vi "ForceAndPressureAhmed.vi"() -> ()   [LabVIEW 2017]
uses:
  <vilib>/Analysis/Matrix/Numeric/Conversions/Matrix To Array - RM.vi
  <vilib>/Analysis/NI_AALBase.lvlib
  <vilib>/Analysis/Matrix/NI_Matrix.lvlib
panel:
  out "Velocity (m/s)":dbl=1.0208025474683848
  out "Force Mean Convergence":dbl(graph)=0.23332198796908798
  out "Pressure Mean Convergence":dbl(graph)=0.00022051026462577283
  in  "Balance Check":i32
  in  "Tapping Check":i32=1
  in  "Comment":string="test"
  in  "Time (s)":dbl=10.0 format="%#_13g"
  in  "Frequency (Hz)":dbl=1000.0 format="%#_13g"
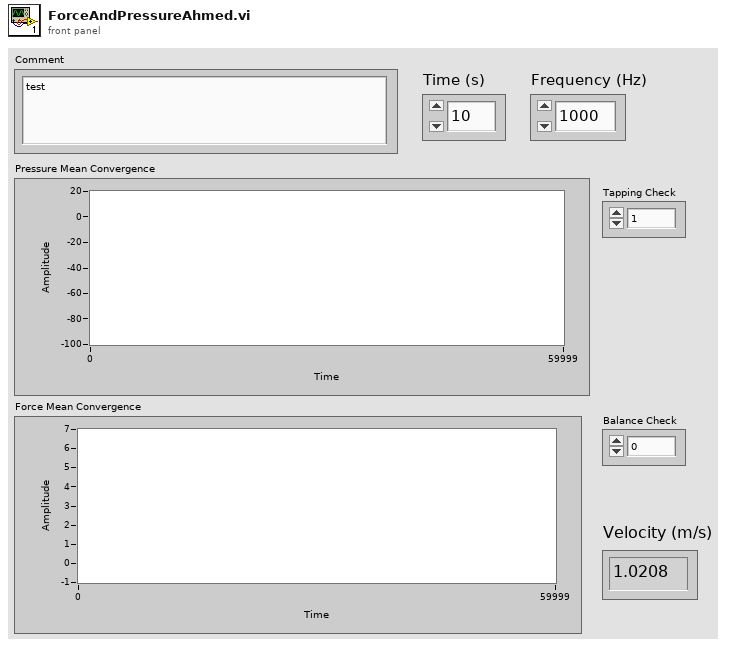
[diagram p1: front panel]
types:
  T1 = typedef "Real Matrix NI_Silver.ctl" = dbl[][]
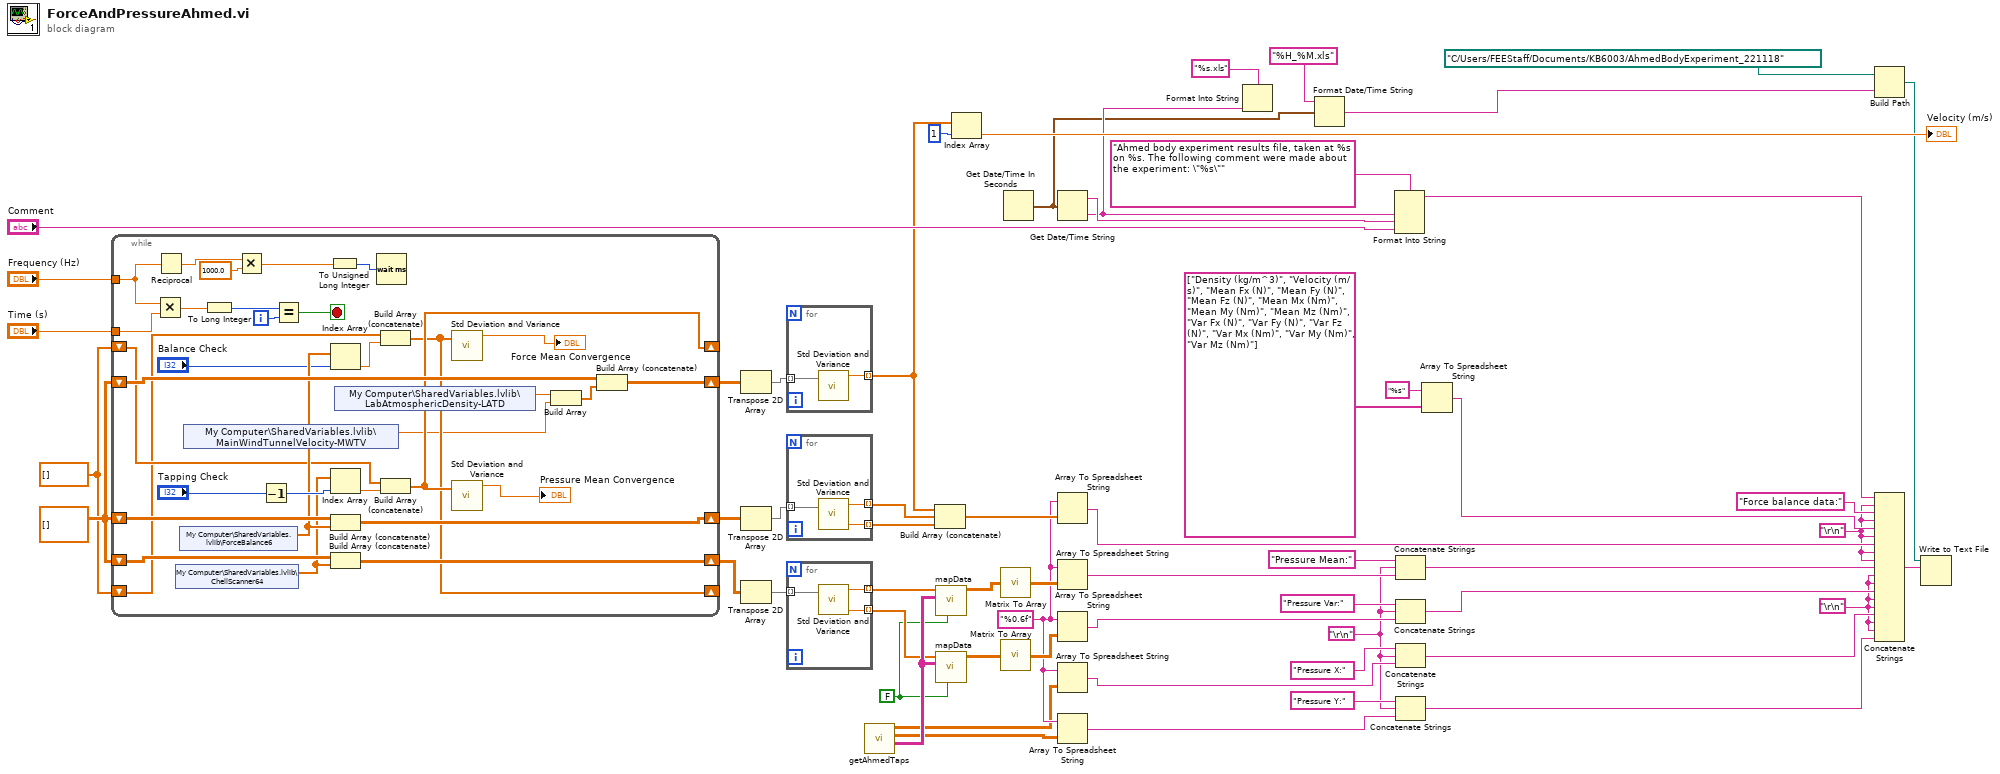
[diagram p0: block diagram]
diagram:
  w15 = dbl[] []
  w20 = "\r\n"
  w24 = "\r\n"
  w12 = "\r\n"
  w35 = "%0.6f" ("format string")
  w50 = FALSE ("Zero Index")
  w46 = dbl[][] []
  n1 = while {
    tunnel: "Frequency (Hz)" -> [w87]
    tunnel: "Time (s)" -> [w86]
    shift-right: [w81] -> w57
    shift-left: w46 -> [w80]
    shift-right: [w82] -> w56
    shift-left: w46 -> [w79]
    shift-right: [w76] -> w45
    shift-left: w46 -> [w75]
    shift-right: [w68] -> _
    shift-left: w15 -> [w70]
    shift-right: [w64] -> _
    shift-left: w15 -> [w66]
    i -> [w69]
    stop <- w83 stop-if-true
    n2 = Multiply(x=w87, y=w86) -> (x*y=w85:dbl)
    n3 = Reciprocal(x=w87) -> (1/x=w91:dbl)
    n4 = shared-variable "My Computer\\SharedVariables.lvlib\\ChellScanner64"() -> (w61:dbl[])  [unwired: 1 in, 1 out]
    n5 = shared-variable "My Computer\\SharedVariables.lvlib\\ForceBalance6"() -> (w72:dbl[])  [unwired: 1 in, 1 out]
    n6 = shared-variable "My Computer\\SharedVariables.lvlib\\MainWindTunnelVelocity-MWTV"() -> (w60:dbl)  [unwired: 1 in, 1 out]
    n7 = To Long Integer(number=w85) -> (32bit integer=w84:i32)
    n8 = Multiply(x=w91, y=1000.0) -> (x*y=w90:dbl)
    n9 = Decrement(x="Tapping Check") -> (x-1=w73:i32)
    n10 = Equal?(x=w84, y=w69) -> (x = y?=w83:bool)
    n11 = To Unsigned Long Integer(number=w90) -> (unsigned 32bit integer=w89:u32)
    n12 = Index Array(array=w72, index="Balance Check") -> (element=w65:dbl)
    n13 = Index Array(array=w61, index=w73) -> (element=w62:dbl)
    n14 = Build Array (concatenate)(w80, w72) -> (w81:dbl[][])
    n15 = Build Array (concatenate)(w79, w61) -> (w82:dbl[][])
    n16 = shared-variable "My Computer\\SharedVariables.lvlib\\LabAtmosphericDensity-LATD"() -> (w78:dbl)  [unwired: 1 in, 1 out]
    n17 = Wait (ms)(milliseconds to wait=w89) -> ()  [unwired: 1 out]
    n18 = Build Array (concatenate)(w66, w65) -> (w64:dbl[])
    n19 = Build Array (concatenate)(w70, w62) -> (w68:dbl[])
    n20 = call <vilib>:"Std Deviation and Variance.vi"("X"=w64) -> ("mean"=→"Force Mean Convergence":dbl)  [unwired: 1 in, 2 out]
    n21 = call <vilib>:"Std Deviation and Variance.vi"("X"=w68) -> ("mean"=→"Pressure Mean Convergence":dbl)  [unwired: 1 in, 2 out]
    n22 = Build Array(w78, w60) -> (w77:dbl[])
    n23 = Build Array (concatenate)(w75, w77) -> (w76:dbl[][])
  }
  n24 = Transpose 2D Array(2D array=w45) -> (transposed array=w44:dbl[][])
  n25 = Transpose 2D Array(2D array=w57) -> (transposed array=w55:dbl[][])
  n26 = Transpose 2D Array(2D array=w56) -> (transposed array=w54:dbl[][])
  n27 = for {
    tunnel: w44 -> [w93] mode=indexing
    tunnel: [w92] -> w10 mode=indexing
    n28 = call <vilib>:"Std Deviation and Variance.vi"("X"=w93) -> ("mean"=w92:dbl)  [unwired: 1 in, 2 out]
  }
  n29 = for {
    tunnel: w55 -> [w96] mode=indexing
    tunnel: [w95] -> w17 mode=indexing
    tunnel: [w94] -> w16 mode=indexing
    n30 = call <vilib>:"Std Deviation and Variance.vi"("X"=w96) -> ("mean"=w95:dbl, "variance"=w94:dbl)  [unwired: 1 in, 1 out]
  }
  n31 = for {
    tunnel: w54 -> [w99] mode=indexing
    tunnel: [w98] -> w53 mode=indexing
    tunnel: [w97] -> w51 mode=indexing
    n32 = call <vilib>:"Std Deviation and Variance.vi"("X"=w99) -> ("mean"=w98:dbl, "variance"=w97:dbl)  [unwired: 1 in, 1 out]
  }
  n33 = call "getAhmedTaps.vi"() -> ("MAP"=w52:string[][], "Y"=w33:dbl[][], "X"=w34:dbl[][])  [unwired: 7 in]
  n34 = Build Array (concatenate)(w10, w17, w16) -> (w47:dbl[])
  n35 = call "mapData.vi"("Zero Index"=w50, "MAP"=w52, "1D Data"=w53) -> ("Real Matrix"=w49:T1)  [unwired: 8 in]
  n36 = call "mapData.vi"("Zero Index"=w50, "MAP"=w52, "1D Data"=w51) -> ("Real Matrix"=w48:T1)  [unwired: 8 in]
  n37 = Index Array(array=w10, index=1) -> (element=→"Velocity (m/s)":dbl)
  n38 = call-poly <vilib>:"Matrix To Array.vi"("Real Matrix"=w49) -> ("Real 2D Array"=w41:dbl[][])
  n39 = call-poly <vilib>:"Matrix To Array.vi"("Real Matrix"=w48) -> ("Real 2D Array"=w40:dbl[][])
  n40 = Get Date/Time In Seconds() -> (seconds since 1Jan1904=w3:timestamp)
  n41 = Get Date/Time String(seconds (now)=w3) -> (date string=w37:string, time string=w7:string)  [unwired: 2 in]
  n42 = Array To Spreadsheet String(array=w47, 3:w35) -> (spreadsheet string=w36:string)  [unwired: 1 in]
  n43 = Array To Spreadsheet String(array=w41, 3:w35) -> (spreadsheet string=w25:string)  [unwired: 1 in]
  n44 = Array To Spreadsheet String(array=w40, 3:w35) -> (spreadsheet string=w27:string)  [unwired: 1 in]
  n45 = Array To Spreadsheet String(array=w34, 3:w35) -> (spreadsheet string=w29:string)  [unwired: 1 in]
  n46 = Array To Spreadsheet String(array=w33, 3:w35) -> (spreadsheet string=w31:string)  [unwired: 1 in]
  n47 = Format Into String(format string="%s.xls" ("initial string"), w7) -> ()  [unwired: 2 in, 2 out]
  n48 = Format Date/Time String(time format string (%c)="%H_%M.xls", seconds (now)=w3) -> (date/time string=w1:string)  [unwired: 1 in]
  n49 = Format Into String(format string="Ahmed body experiment results file, taken at %s on %s. The following comment were made about the experiment: \"%s\"", w7, w37, "Comment") -> (resulting string=w11:string)  [unwired: 2 in, 1 out]
  n50 = Concatenate Strings("Pressure Mean:" ("string"), w24, w25) -> (w23:string)
  n51 = Concatenate Strings("Pressure Var:" ("string"), w24, w27) -> (w22:string)
  n52 = Concatenate Strings("Pressure X:" ("string"), w24, w29) -> (w21:string)
  n53 = Concatenate Strings("Pressure Y:" ("string"), w24, w31) -> (w19:string)
  n54 = Array To Spreadsheet String(array=string[] ["Density (kg/m^3)", "Velocity (m/s)", "Mean Fx (N)", "Mean Fy (N)", "Mean Fz (N)", "Mean Mx (Nm)", "Mean My (Nm)", "Mean Mz (Nm)", "Var Fx (N)", "Var Fy (N)", "Var Fz (N)", "Var Mx (Nm)", "Var My (Nm)", "Var Mz (Nm)"], 3:"%s" ("format string")) -> (spreadsheet string=w14:string)  [unwired: 1 in]
  n55 = Build Path(base path=path "C:/Users/FEEStaff/Documents/KB6003/AhmedBodyExperiment_221118" ("file (use dialog)"), name or relative path=w1) -> (appended path=w5:path)
  n56 = Concatenate Strings(w11, w12, "Force balance data:" ("string"), w12, w14, w12, w36, w12, w12, w23, w20, w20, w22, w20, w20, w21, w20, w20, w19) -> (w18:string)
  n57 = Write to Text File(file (use dialog)=w5, text=w18) -> ()  [unwired: 2 in, 3 out]
